vi "Resize Data Row Options.vi"(10 "number of data rows (1)":i32=1, 11 "draw options in":T1={"Background Color"=16777215, "Grid Color"=13816530, "Angle Units"=enum."Radians", "Draw Solid Background"=TRUE, "Draw Grid"=TRUE, "Grid Spacing"=1.0, "AutoScale"=TRUE, "Fit to Radius"=1.0, "data row options"=[]}) -> (3 "draw options out":T1={"Background Color"=16777215, "Grid Color"=13816530, "Angle Units"=enum."Radians", "Draw Solid Background"=TRUE, "Draw Grid"=TRUE, "Grid Spacing"=1.0, "AutoScale"=TRUE, "Fit to Radius"=1.0, "data row options"=[]})   [LabVIEW 2017, in "NI_Robotics_2D Rangefinder Picture.lvlib"]
uses:
  <vilib>/robotics/Controls/2D Rangefinder/2D Rangefinder Picture/NI_Robotics_2D Rangefinder Picture.lvlib
  <vilib>/robotics/Controls/2D Rangefinder/2D Rangefinder Picture/Draw Options.ctl
  <vilib>/robotics/Controls/Utilities/Angle Units.ctl
  <vilib>/robotics/Controls/2D Rangefinder/2D Rangefinder Picture/Data Row Options.ctl
  <vilib>/robotics/Controls/Utilities/NI_Robotics_Control Utilities.lvlib
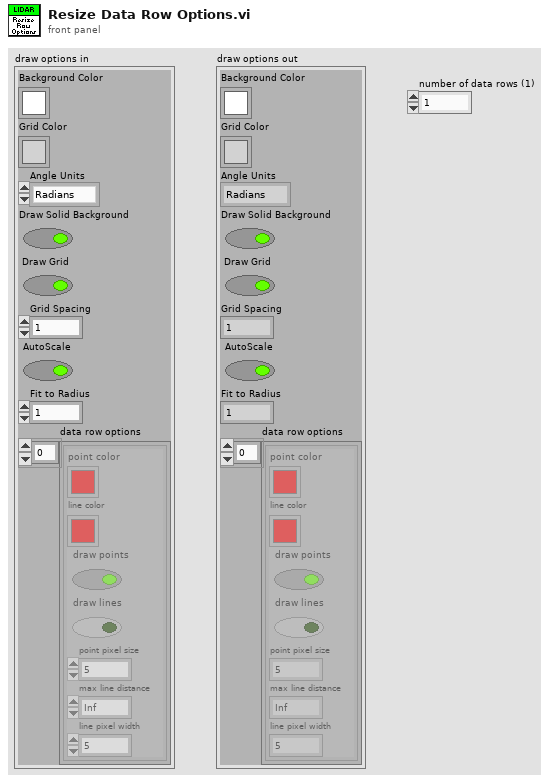
[diagram p1: front panel]
types:
  T1 = typedef "NI_Robotics_2D Rangefinder Picture.lvlib/Draw Options.ctl" = cluster{"Background Color":u32, "Grid Color":u32, "Angle Units":T2, "Draw Solid Background":bool, "Draw Grid":bool, "Grid Spacing":dbl, "AutoScale":bool, "Fit to Radius":dbl, "data row options":T3[]}
  T2 = typedef "NI_Robotics_Control Utilities.lvlib/Angle Units.ctl" = enum16{"Radians", "Degrees"}
  T3 = typedef "NI_Robotics_2D Rangefinder Picture.lvlib/Data Row Options.ctl" = cluster{"point color":u32, "line color":u32, "draw points":bool, "draw lines":bool, "point pixel size":u16, "max line distance":dbl, "line pixel width":u16}
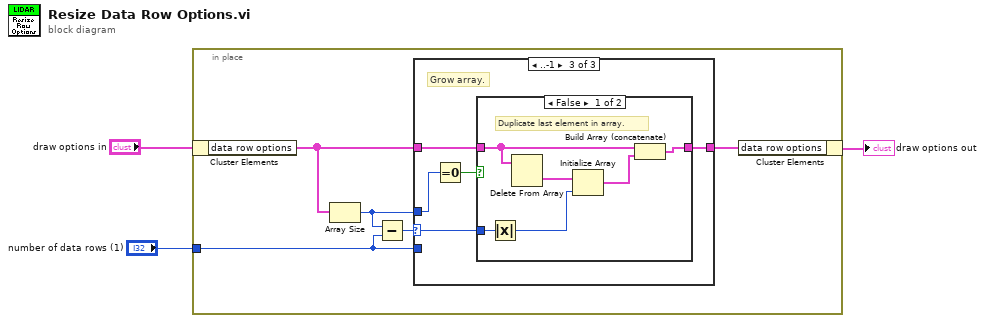
[diagram p0: block diagram]
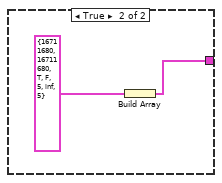
[diagram p4: hidden frame]
diagram:
  n1 = in-place {
    in-place-border: "number of data rows (1)" -> [w5]
    n2 = in-place-cluster #1("draw options in") -> ("data row options"=w8:T3[])
    n3 = Array Size(array=w8) -> (size(s)=w6:i32)
    n4 = Subtract(x=w6, y=w5) -> (x-y=w4:i32)
    n5 = case shown="..-1" w4 {
      selector: w4 -> [_ _ w11]
      tunnel: w8 -> [w9 w10 w14]
      tunnel: [w9 w10 w12] -> w7
      tunnel: w6 -> [_ _ w13]
      tunnel: w5 -> [_ _ _]
      frame 0, Default {
        # "Same size.  Do nothing."
      }
      frame 1.. {
        # "Do not shrink array."
      }
      frame ..-1 {
        # "Grow array."
        n6 = Equal To 0?(x=w13) -> (x = 0?=w15:bool)
        n7 = case shown="False" w15 {
          tunnel: w14 -> [w20 _]
          tunnel: [w21 w22] -> w12
          tunnel: w11 -> [w18 _]
          frame False {
            # "Duplicate last element in array."
            n8 = Absolute Value(x=w18) -> (abs(x)=w17:i32)
            n9 = Delete From Array(array=w20) -> (deleted portion=w19:T3)  [unwired: 2 in, 1 out]
            n10 = Initialize Array(w19, w17) -> (w16:T3[])
            n11 = Build Array (concatenate)(w20, w16) -> (w21:T3[])
          }
          frame True {
            n12 = Build Array(T3 {"point color"=16711680, "line color"=16711680, "draw points"=TRUE, "draw lines"=FALSE, "point pixel size"=5, "max line distance"=inf, "line pixel width"=5} ("data row options")) -> (w22:T3[])
          }
        }
      }
    }
    n13 = in-place-cluster #1("data row options"=w7) -> (→"draw options out":T1)
  }
